vi "Initialize.vi"(7 "Intent mode":T1, 8 "error in (no error)":errorcluster, 9 "Function Enqueuer":refnum<class "Message Enqueuer.lvclass">, 10 "Array of Hardware":refnum<class "Hardware.lvclass">[](array[class]), 11 "Motions in":refnum<class "Motions.lvclass">) -> (0 "error out":errorcluster, 3 "Motions out":refnum<class "Motions.lvclass">)   [LabVIEW 2016, in "Hardware.lvlib" / "Motions.lvlib" / "Motions.lvclass"]
uses:
  <userlib>/Common Components/Hardware/Abstract System/Motions/Motions/Motions.lvclass
  <userlib>/Common Components/Hardware/Abstract Hardware/Hardware.lvclass
  <vilib>/ActorFramework/Message Enqueuer/Message Enqueuer.lvclass
  <userlib>/Common Components/Hardware/Abstract System/Motions/Motions/Intent_Mode.ctl
  <userlib>/Common Components/TriggerAction Q/TriggerAction Q/TriggerAction Q.lvclass
  <userlib>/Common Components/Hardware/Motor/Motor/Motor.lvclass
  C:/Program Files (x86)/National Instruments/LabVIEW 2016/user.lib/Common Components/Hardware/Abstract Hardware/Hardware.lvclass
  <userlib>/Common Components/Hardware/Abstract System/Motions/Motions/Motor States.ctl
  <userlib>/Common Components/Hardware/Abstract System/Motions/Motions/Intent_Mode_data_UFO.ctl
  <userlib>/Common Components/Hardware/Abstract Hardware/Hardware.lvclass/Hardware.ctl
  <userlib>/Common Components/Hardware/Abstract System/Motions/Motions/Motions.lvclass/Motions.ctl
  <userlib>/Common Components/Hardware/Abstract Hardware/Read Label.vi
  <vilib>/addons/_JKI.lib/Serialization/JSON/JKI JSON Serialization.lvlib
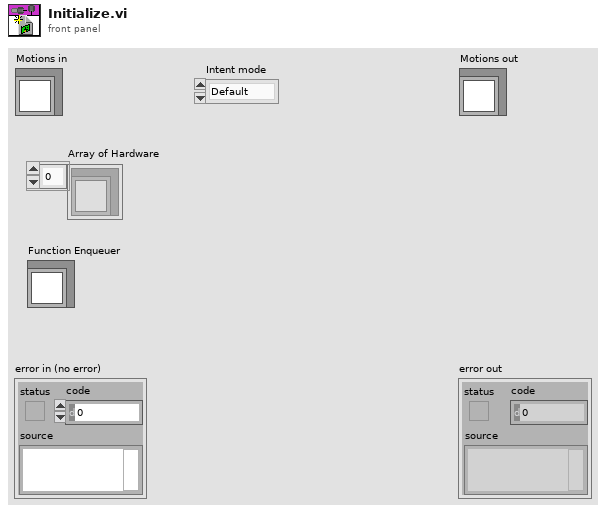
[diagram p1: front panel]
types:
  T1 = typedef "Hardware.lvlib/Motions.lvlib/Motions.lvclass/Intent_Mode.ctl" = enum16{"Default", "XYZ", "UFO"}
  T2 = typedef "Hardware.lvlib/Motions.lvlib/Motions.lvclass/Motor States.ctl" = cluster{"Connected":bool, "Enabled":bool, "Moving Status":bool, "Soft Moving Status":bool, "Current Pos":dbl, "Target Pos":dbl, "Moving Dir (-1, 0, 1)":i32, "Error Status":bool, "Hard Limit+":bool, "Hard Limit-":bool, "Soft Limit+":bool, "Soft Limit-":bool, "History Dst Stack":refnum<queue>, "Motion Status":bool, "Motion TriggerAction Obj":refnum<class "TriggerAction Q.lvclass">, "Jogging":bool}
  T3 = typedef "Hardware.lvlib/Motions.lvlib/Motions.lvclass/Intent_Mode_data_UFO.ctl" = cluster{"ROT":u8, "LIN":u8}
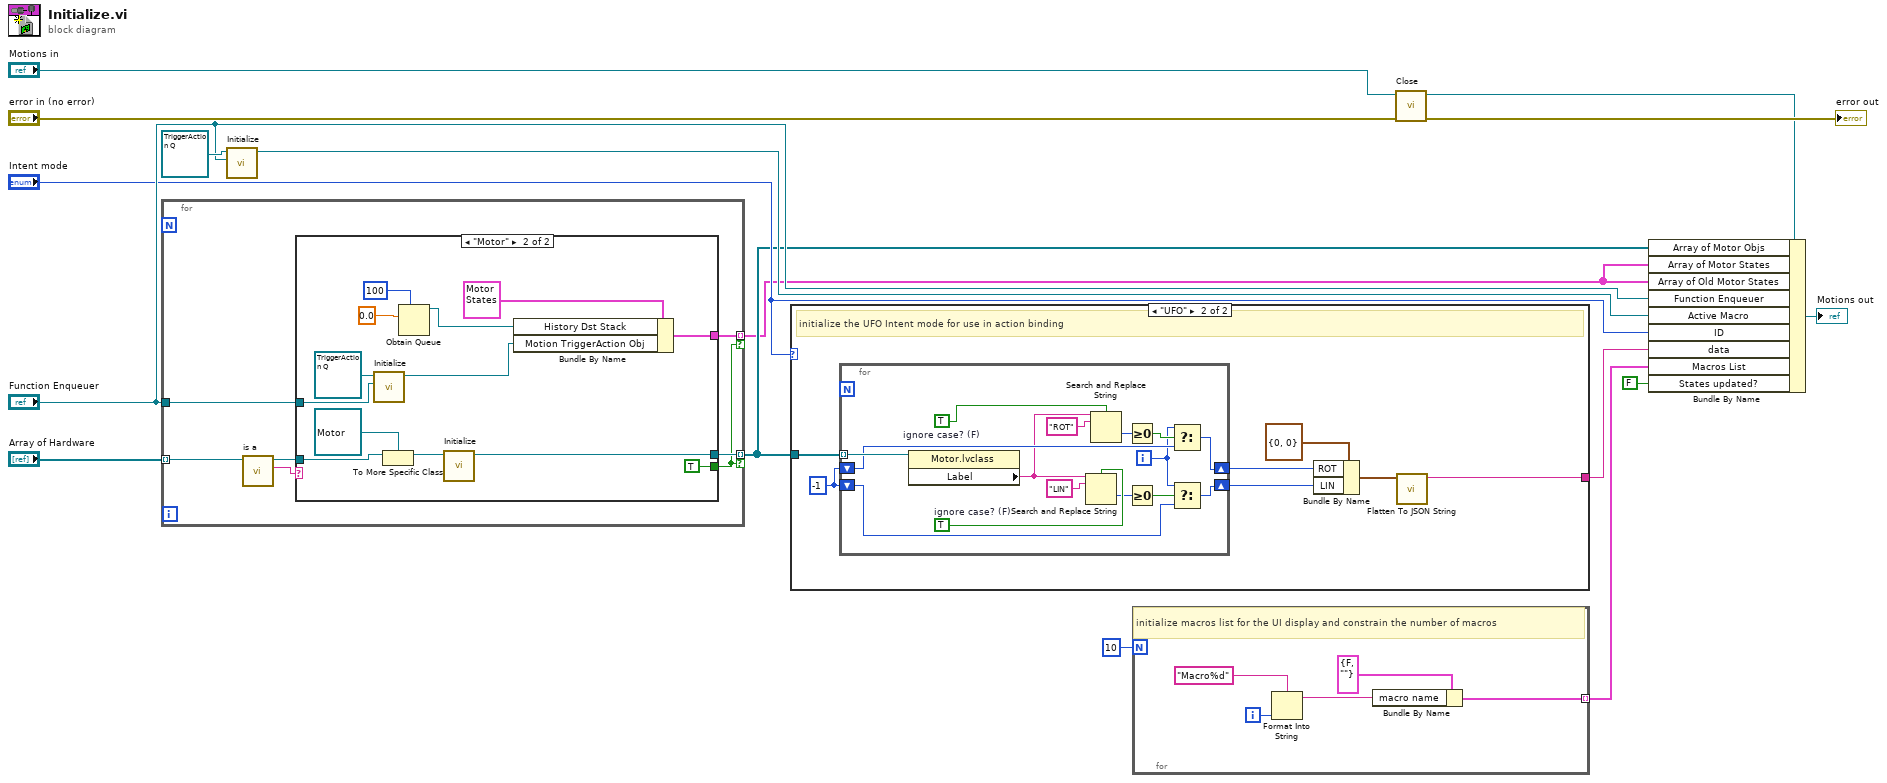
[diagram p0: block diagram]
diagram:
  n1 = for {
    tunnel: "Array of Hardware" -> [w23] mode=indexing
    tunnel: [w20] -> w6 mode=indexing if=w18
    tunnel: [w19] -> w1 mode=indexing if=w18
    tunnel: "Function Enqueuer" -> [w17]
    n2 = call-dynamic "is a.vi"("Hardware in"=w23) -> ("is a"=w22:string, "Hardware out"=w21:refnum<class "Hardware.lvclass">)  [unwired: 8 in, 1 out]
    n3 = case shown="\"Motor\"" w22 {
      tunnel: w21 -> [_ w31]
      tunnel: [_ w24] -> w20
      tunnel: [_ TRUE] -> w18
      tunnel: [_ w32] -> w19
      tunnel: w17 -> [_ w25]
      frame Default {
      }
      frame "Motor" {
        n4 = call <userlib>:"Initialize.vi"("Function Enqueuer"=w25, "TriggerAction in"=refnum<class "TriggerAction Q.lvclass"> refnum ("TriggerAction.lvclass")) -> ("TriggerAction out"=w26:refnum<class "TriggerAction Q.lvclass">)  [unwired: 8 in, 1 out]
        n5 = To More Specific Class(target class=refnum<class "Motor.lvclass"> refnum ("Hardware.lvlib:Motor.lvlib:Motor.lvclass"), reference=w31) -> (specific class reference=w35:refnum<class "Motor.lvclass">)  [unwired: 1 in, 1 out]
        n6 = Obtain Queue(max queue size (-1, unlimited)=100, element data type=0.0) -> (queue out=w29:refnum<queue>)  [unwired: 3 in, 2 out]
        n7 = call-dynamic <userlib>:"Initialize.vi"("CCD in"=w35) -> ("CCD out"=w24:refnum<class "Motor.lvclass">)  [unwired: 9 in, 1 out]
        n8 = Bundle By Name(cluster=T2 {"Connected"=FALSE, "Enabled"=FALSE, "Moving Status"=FALSE, "Soft Moving Status"=FALSE, "Current Pos"=0.0, "Target Pos"=0.0, "Moving Dir (-1, 0, 1)"=0, "Error Status"=FALSE, "Hard Limit+"=FALSE, "Hard Limit-"=FALSE, "Soft Limit+"=FALSE, "Soft Limit-"=FALSE, "History Dst Stack"=refnum, "Motion Status"=FALSE, "Motion TriggerAction Obj"=refnum, "Jogging"=FALSE} ("Cluster"), "History Dst Stack"=w29, "Motion TriggerAction Obj"=w26) -> (w32:T2)
      }
    }
  }
  n9 = call <userlib>:"Initialize.vi"("Function Enqueuer"="Function Enqueuer", "TriggerAction in"=refnum<class "TriggerAction Q.lvclass"> refnum ("TriggerAction.lvclass")) -> ("TriggerAction out"=w8:refnum<class "TriggerAction Q.lvclass">)  [unwired: 8 in, 1 out]
  n10 = case shown="\"UFO\"" "Intent mode" {
    tunnel: w6 -> [_ w42]
    tunnel: [_ w37] -> w5
    frame Default {
    }
    frame "UFO" {
      w41 = -1
      # "initialize the UFO Intent mode for use in action binding"
      n11 = for {
        tunnel: w42 -> [w58] mode=indexing
        shift-right: [w54] -> w40
        shift-left: w41 -> [w52]
        shift-right: [w44] -> w39
        shift-left: w41 -> [w46]
        i -> [w45]
        w50 = TRUE  # ignore case? (F)
        w56 = TRUE  # ignore case? (F)
        n12 = property class="Motor.lvclass"(reference=w58) -> ("Label"=w47:string)  [unwired: 1 in, 2 out]
        n13 = Search and Replace String(case sensitive?=w50, input string=w47, search string="LIN") -> (offset past replacement=w49:i32)  [unwired: 5 in, 3 out]
        n14 = Search and Replace String(case sensitive?=w56, input string=w47, search string="ROT") -> (offset past replacement=w55:i32)  [unwired: 5 in, 3 out]
        n15 = Greater Or Equal To 0?(x=w55) -> (x >= 0?=w53:bool)
        n16 = Greater Or Equal To 0?(x=w49) -> (x >= 0?=w48:bool)
        n17 = Select(t=w45, s=w53, f=w52) -> (s? t:f=w54:i32)
        n18 = Select(t=w45, s=w48, f=w46) -> (s? t:f=w44:i32)
      }
      n19 = Bundle By Name(cluster=T3 {"ROT"=0, "LIN"=0} ("UFO Intent Mode data"), "ROT"=w40, "LIN"=w39) -> (w38:T3)
      n20 = call <vilib>:"Flatten To JSON String.vi"("Variant"=w38) -> ("JSON String"=w37:string)  [unwired: 9 in, 1 out]
    }
  }
  n21 = for {
    N: 10 -> [_]
    tunnel: [w59] -> w3 mode=indexing
    i -> [w61]
    # "initialize macros list for the UI display and constrain the number of macros"
    n22 = Format Into String(format string="Macro%d", w61) -> (resulting string=w60:string)  [unwired: 2 in, 1 out]
    n23 = Bundle By Name(cluster=cluster{"enabled?":bool, "macro name":string} {"enabled?"=FALSE, "macro name"=""} ("Cluster"), "macro name"=w60) -> (w59:cluster{"enabled?":bool, "macro name":string})
  }
  n24 = call <userlib>:"Close.vi"("error in (no error)"="error in (no error)", "Motions in"="Motions in") -> ("error out"=→"error out":errorcluster, "Motions out"=w12:refnum<class "Motions.lvclass">)  [unwired: 8 in]
  n25 = Bundle By Name(cluster=w12, "Array of Motor Objs"=w6, "Array of Motor States"=w1, "Array of Old Motor States"=w1, "Function Enqueuer"="Function Enqueuer", "Active Macro"=w8, "ID"="Intent mode", "data"=w5, "Macros List"=w3, "States updated?"=FALSE ("States valid?")) -> (→"Motions out":refnum<class "Motions.lvclass">)
